vi "Setup APU 1.3.vi"(5 "acceleration (RPM/sec) (0)":dbl, 6 "event stuck limit (ms) (200)":dbl=200.0, 7 "enable acceleration (F)":bool, 8 "error in (no error)":errorcluster, 9 "start position (deg) (0)":dbl, 10 "speed (RPM) (0)":dbl, 11 "APU in":refnum<class "APU.lvclass">) -> (0 "error out":errorcluster, 3 "APU out":refnum<class "APU.lvclass">)   [LabVIEW 2013, in "APU.lvclass"]
uses:
  APU.lvclass
  Engine Simulation IP.lvclass/Engine Simulation IP.ctl
  APU.lvclass/APU.ctl
  <vilib>/NI/LVFPGA Adv Session Resources/OpenByNameSubVI.vi
  <vilib>/rvi/interface/common/dynamic/niFpgaEscapeDelimiterAndNull.vi
  <vilib>/Utility/error.llb/Error Cluster From Error Code.vi
  <vilib>/rvi/interface/common/niFpgaWaitOnOcc.vi
  <vilib>/rvi/errors/niLvFpgaAdjustHostInterfaceError.vi
  <vilib>/FPGAPlugInAG/Dynamic/niLvFpga_Close_Dynamic.vi
  <vilib>/NI/LVFPGA Adv Session Resources/OpenByName.xnode
  <vilib>/rvi/interface/nirviReadWriteControl/nirviReadWriteControl.xnode
  <vilib>/rvi/interface/nirviCloseFPGA/nirviCloseFPGA.xnode
  Engine Simulation IP.lvclass
  <vilib>/NI/LVFPGA Adv Session Resources/LVFPGAAdvSessionResources.lvlib
  NiFpgaLv.dll
  <vilib>/rvi/interface/Simulation/niFpgaSimulationCallBeginRW.vi
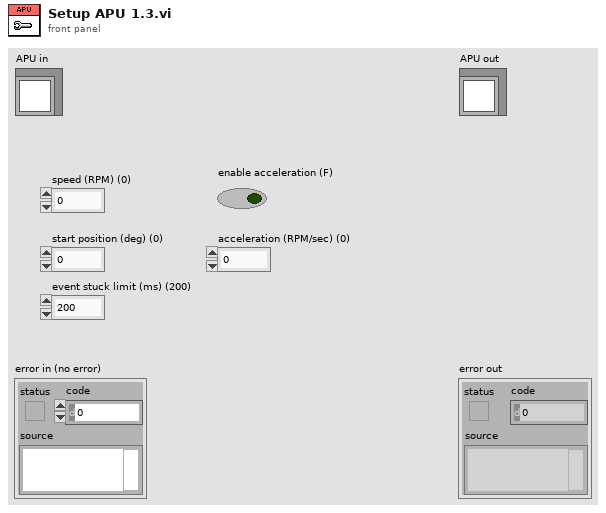
[diagram p1: front panel]
types:
  T1 = cluster{"desired speed":fxp<+/-,23,2>, "reset":bool}
  T2 = cluster{"acceleration":fxp<+,18,-20>, "enable accel":bool}
  T3 = cluster{"start":fxp<+,17,17>, "stuck limit":fxp<+,18,18>}
  T4 = cluster{"Name":string, "Depth":u32, "Write? (Deprecated:Use Implementation)":bool, "Physical Channel":u32, "Base Address":u32, "Data Width":u32, "Data Type":enum32{"Boolean", "I8", "I16", "I32", "I64", "U8", "U16", "U32", "U64", "FXP", "CustomControl", "SGL"}, "FXP Properties":variant, "Write Window Address":u32, "Implementation":enum16{"niFpgaTargetToHost", "niFpgaHostToTarget", "niFpgaPeerToPeerWriter", "niFpgaPeerToPeerReader", "niCoreTargetToHost", "niCoreHostToTarget"}, "Control Set":u32}[]
  T5 = cluster{"Name":string, "type":variant, "indicator?":bool}[]
  T6 = typedef "Engine Simulation Session.lvclass/Bitfile Major Version.ctl" = enum16{"1.0", "1.1", "1.2", "1.3"}
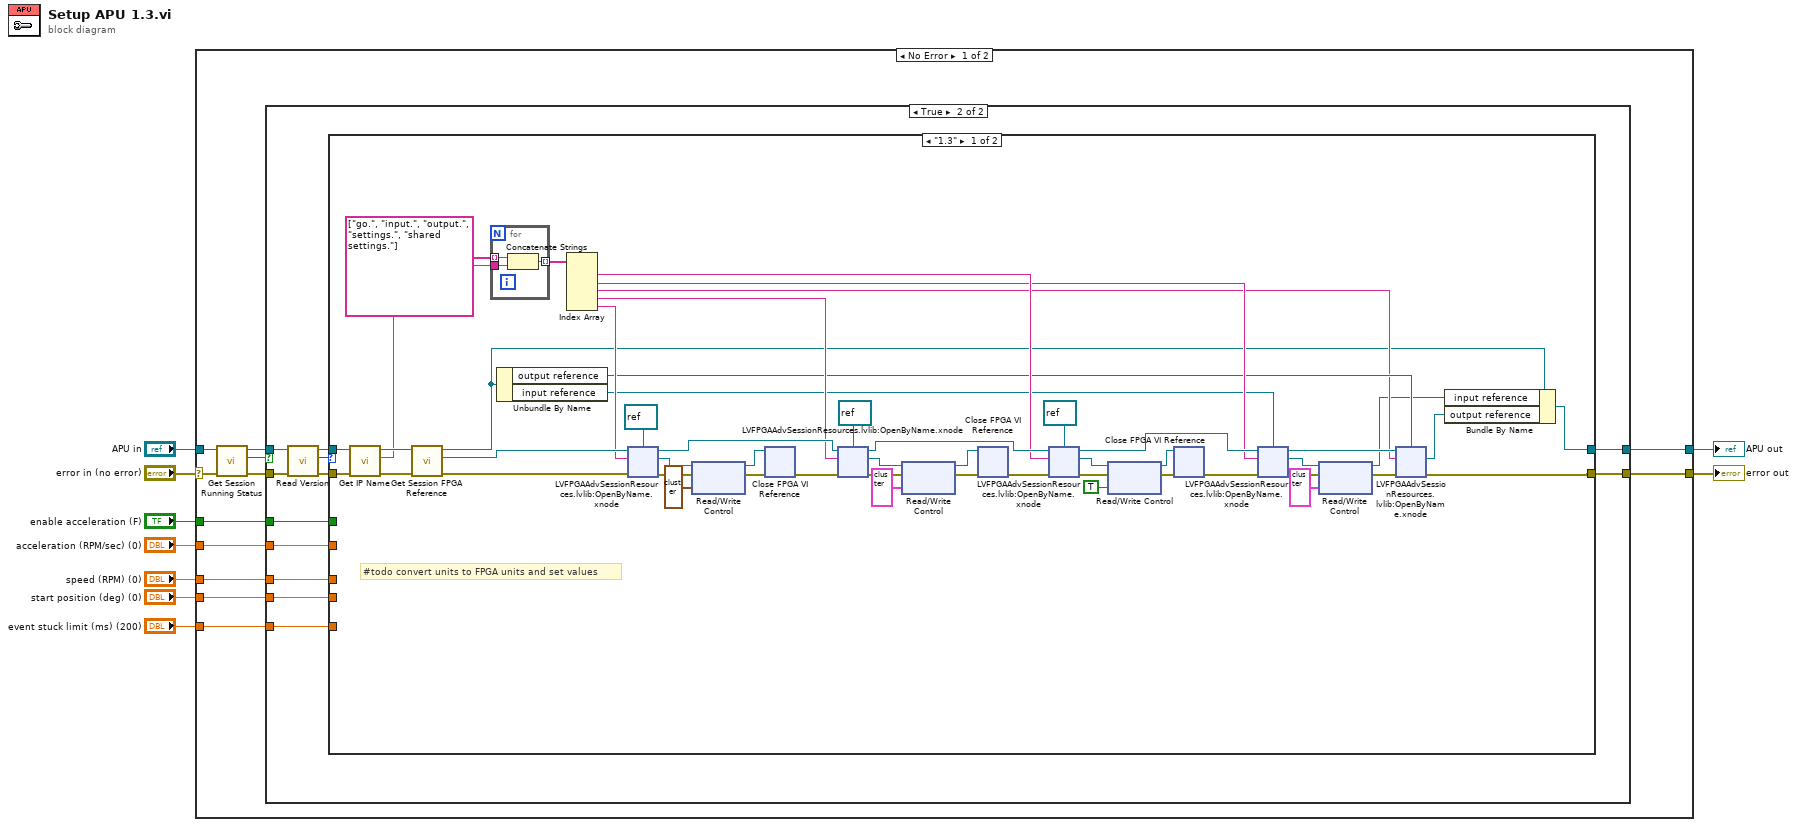
[diagram p0: block diagram]
diagram:
  n1 = case shown="No Error" "error in (no error)" {
    selector: "error in (no error)" -> [w21 w157]
    tunnel: [w18 w157] -> w8
    tunnel: [w15 w156] -> w6
    tunnel: "APU in" -> [w20 w156]
    tunnel: "enable acceleration (F)" -> [w14 _]
    tunnel: "acceleration (RPM/sec) (0)" -> [w13 _]
    tunnel: "speed (RPM) (0)" -> [w12 _]
    tunnel: "start position (deg) (0)" -> [w11 _]
    tunnel: "event stuck limit (ms) (200)" -> [w10 _]
    frame No Error {
      n2 = call "Get Session Running Status.vi"("error in (no error)"=w21, "Engine Simulation IP in"=w20) -> ("error out"=w17:errorcluster, "running"=w19:bool, "Engine Simulation IP out"=w16:refnum<class "APU.lvclass">)  [unwired: 7 in]
      n3 = case shown="True" w19 {
        tunnel: [w23 w33] -> w18
        tunnel: w17 -> [w23 w35]
        tunnel: w16 -> [w22 w34]
        tunnel: [w22 w29] -> w15
        tunnel: w14 -> [_ w28]
        tunnel: w13 -> [_ w27]
        tunnel: w12 -> [_ w26]
        tunnel: w11 -> [_ w25]
        tunnel: w10 -> [_ w24]
        frame False {
          # "#todo throw not running error"
        }
        frame True {
          n4 = call "Read Version.vi"("error in (no error)"=w35, "Engine Simulation IP in"=w34) -> ("error out"=w32:errorcluster, "version"=w31:T6, "Engine Simulation IP out"=w30:refnum<class "APU.lvclass">)  [unwired: 7 in]
          n5 = case shown="\"1.3\"" w31 {
            tunnel: [w42 w155] -> w33
            tunnel: w32 -> [w63 w155]
            tunnel: w30 -> [w62 w154]
            tunnel: [w41 w154] -> w29
            tunnel: w28 -> [_ _]
            tunnel: w27 -> [_ _]
            tunnel: w26 -> [_ _]
            tunnel: w25 -> [_ _]
            tunnel: w24 -> [_ _]
            frame "1.3" {
              # "#todo convert units to FPGA units and set values"
              n6 = call "Get IP Name.vi"("error in (no error)"=w63, "Engine Simulation IP in"=w62) -> ("error out"=w60:errorcluster, "Name"=w58:string, "Engine Simulation IP out"=w61:refnum<class "APU.lvclass">)  [unwired: 7 in]
              n7 = call "Get Session FPGA Reference.vi"("error in (no error)"=w60, "Engine Simulation IP in"=w61) -> ("error out"=w65:errorcluster, "fpga reference"=w64:refnum<k20>, "Engine Simulation IP out"=w43:refnum<class "APU.lvclass">)  [unwired: 7 in]
              n8 = for {
                tunnel: w58 -> [w114]
                tunnel: string[] ["go.", "input.", "output.", "settings.", "shared settings."] -> [w113] mode=indexing
                tunnel: [w112] -> w57 mode=indexing
                n9 = Concatenate Strings(w113, w114) -> (w112:string)
              }
              n10 = Unbundle By Name(w43) -> ("output reference"=w45:refnum<k20>, "input reference"=w46:refnum<k20>)
              n11 = Index Array(array=w57) -> (element #1=w54:string, element #2=w47:string, element #3=w44:string, element #4=w55:string, element #5=w56:string)  [unwired: 5 in]
              n12 = xnode "LVFPGAAdvSessionResources.lvlib:OpenByName.xnode"("FPGA VI Reference in"=w64, "Resource name in"=w56, "Single resource reference type in"=refnum<k20> refnum ("shared settings"), "Error in"=w65) -> ("Single resource reference out"=w68:refnum<k20>, "Error out"=w66:errorcluster, "FPGA VI Reference out"=w74:refnum<k20>)
              n13 = xnode "Read/Write Control"("FPGA VI Reference In"=w68, "error in"=w66, "Value"=T3 {"start"=0.0, "stuck limit"=0.0}) -> ("FPGA VI Reference Out"=w73:refnum<k20>, "error out"=w71:errorcluster)
              n14 = xnode "Close FPGA VI Reference"("FPGA VI Reference In"=w73, "error in"=w71) -> ("error out"=w72:errorcluster)
              n15 = xnode "LVFPGAAdvSessionResources.lvlib:OpenByName.xnode"("FPGA VI Reference in"=w74, "Resource name in"=w55, "Single resource reference type in"=refnum<k20> refnum ("apu settings"), "Error in"=w72) -> ("Single resource reference out"=w69:refnum<k20>, "Error out"=w70:errorcluster, "FPGA VI Reference out"=w80:refnum<k20>)
              n16 = xnode "Read/Write Control"("FPGA VI Reference In"=w69, "error in"=w70, "Value"=T2 {"acceleration"=0.0, "enable accel"=FALSE}) -> ("FPGA VI Reference Out"=w77:refnum<k20>, "error out"=w76:errorcluster)
              n17 = xnode "Close FPGA VI Reference"("FPGA VI Reference In"=w77, "error in"=w76) -> ("error out"=w78:errorcluster)
              n18 = xnode "LVFPGAAdvSessionResources.lvlib:OpenByName.xnode"("FPGA VI Reference in"=w80, "Resource name in"=w54, "Single resource reference type in"=refnum<k20> refnum ("go reference"), "Error in"=w78) -> ("Single resource reference out"=w83:refnum<k20>, "Error out"=w79:errorcluster, "FPGA VI Reference out"=w48:refnum<k20>)
              n19 = xnode "Read/Write Control"("FPGA VI Reference In"=w83, "error in"=w79, "Value"=TRUE) -> ("FPGA VI Reference Out"=w85:refnum<k20>, "error out"=w82:errorcluster)
              n20 = xnode "Close FPGA VI Reference"("FPGA VI Reference In"=w85, "error in"=w82) -> ("error out"=w49:errorcluster)
              n21 = xnode "LVFPGAAdvSessionResources.lvlib:OpenByName.xnode"("FPGA VI Reference in"=w48, "Resource name in"=w47, "Single resource reference type in"=w46, "Error in"=w49) -> ("Single resource reference out"=w52:refnum<k20>, "Error out"=w51:errorcluster, "FPGA VI Reference out"=w50:refnum<k20>)
              n22 = xnode "Read/Write Control"("FPGA VI Reference In"=w52, "error in"=w51, "Value"=T1 {"desired speed"=0.0, "reset"=FALSE}) -> ("FPGA VI Reference Out"=w36:refnum<k20>, "error out"=w53:errorcluster)
              n23 = xnode "LVFPGAAdvSessionResources.lvlib:OpenByName.xnode"("FPGA VI Reference in"=w50, "Resource name in"=w44, "Single resource reference type in"=w45, "Error in"=w53) -> ("Single resource reference out"=w37:refnum<k20>, "Error out"=w42:errorcluster)  [unwired: 1 out]
              n24 = Bundle By Name(cluster=w43, "input reference"=w36, "output reference"=w37) -> (w41:refnum<class "APU.lvclass">)
            }
            frame Default {
              # "#todo throw wrong version error"
            }
          }
        }
      }
    }
    frame Error {
    }
  }
  "error out" <- w8
  "APU out" <- w6
